vi "Mutate 1.3.3.vi"(8 "error in (no error)":errorcluster, 11 "Device Ref in":T1 format="%.0x") -> (0 "error out":errorcluster, 3 "Device Ref out":T1 format="%.0x")   [LabVIEW 2015, in "Engine Simulation Toolkit System Explorer.lvlib"]
uses:
  Engine Simulation Toolkit System Explorer.lvlib
  <vilib>/NI Veristand/Custom Device API/Custom Device Item Ref.ctl
  <vilib>/NI Veristand/Custom Device Tools/Custom Device Utility Library/NI VeriStand - Search for All Items by GUID.vi
  <vilib>/NI Veristand/Custom Device Tools/Custom Device Utility Library/NI VeriStand - Search for Item by Name.vi
  <vilib>/NI VeriStand/Custom Device Tools/Custom Device Utility Library/Custom Device Utility Library.lvlib
  <vilib>/NI VeriStand/Custom Device API/Custom Device API.lvlib
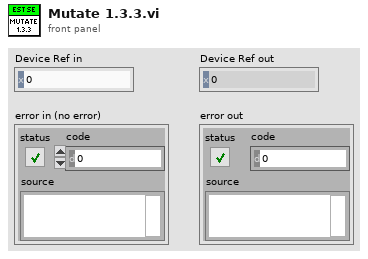
[diagram p1: front panel]
types:
  T1 = typedef "Custom Device API.lvlib/Custom Device Item Ref.ctl" = u64
  T2 = typedef "Engine Simulation Toolkit Shared.lvlib/Channel.ctl" = cluster{"Name":string, "Units":string, "Default":dbl, "Description":string, "Scalable":bool}
  T3 = cluster{"GUID.Status":string, "ChanList.Status Chans":T2[]}[]
  T4 = typedef "Custom Device API.lvlib/Custom Device Item Info.ctl" = cluster{"Name":string, "Is Channel":bool, "GUID":string, "Is Waveform":bool}
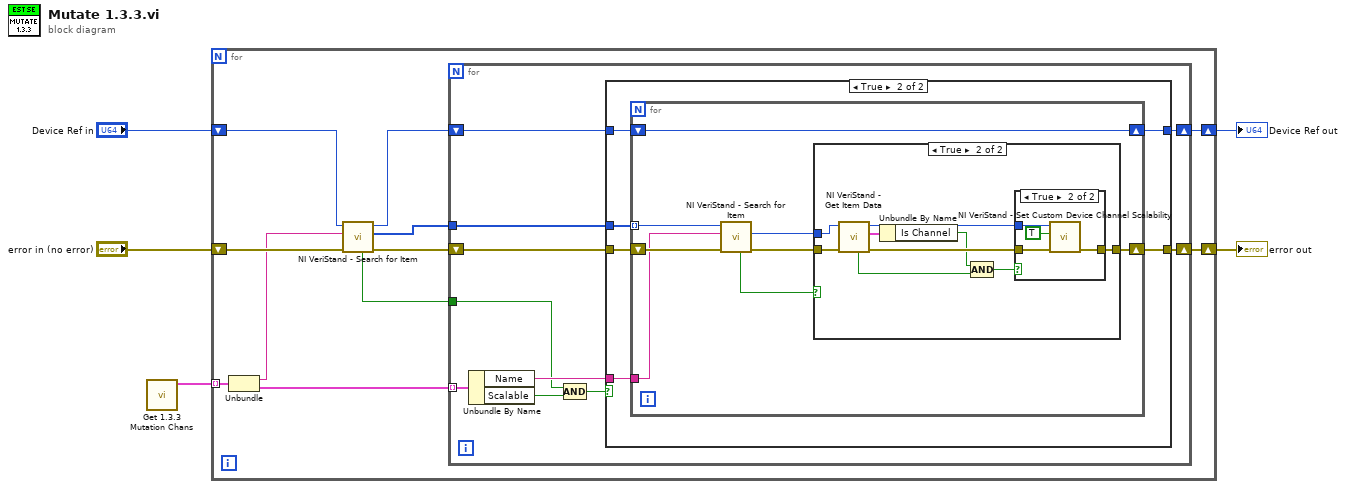
[diagram p0: block diagram]
diagram:
  n1 = call "Get 1.3.3 Mutation Chans.vi"() -> ("Array"=w1:T3)  [unwired: 11 in]
  n2 = for {
    shift-right: [w15] -> w5
    shift-left: "Device Ref in" -> [w16]
    shift-right: [w13] -> w4
    shift-left: "error in (no error)" -> [w14]
    tunnel: w1 -> [w8] mode=indexing
    n3 = Unbundle(w8) -> ("GUID.Status"=w6:string, "ChanList.Status Chans"=w7:T2[])
    n4 = call-poly <vilib>:"NI VeriStand - Search for Item.vi"("error in"=w14, "Item GUID"=w6, "Section Ref in"=w16) -> ("error out"=w9:errorcluster, "Item Refs"=w12:T1[], "Section Ref out"=w10:T1, "Found"=w11:bool)  [unwired: 5 in]
    n5 = for {
      tunnel: w7 -> [w24] mode=indexing
      tunnel: w12 -> [w22]
      tunnel: w11 -> [w18]
      shift-right: [w26] -> w15
      shift-left: w10 -> [w21]
      shift-right: [w25] -> w13
      shift-left: w9 -> [w20]
      n6 = Unbundle By Name(w24) -> ("Name"=w23:string, "Scalable"=w19:bool)
      n7 = Compound Arithmetic op=AND(w18, w19) -> (w17:bool)
      n8 = case shown="True" w17 {
        tunnel: [w28 w29] -> w26
        tunnel: w20 -> [w27 w34]
        tunnel: [w27 w33] -> w25
        tunnel: w23 -> [_ w32]
        tunnel: w22 -> [_ w31]
        tunnel: w21 -> [w28 w30]
        frame False {
        }
        frame True {
          n9 = for {
            tunnel: w32 -> [w38]
            tunnel: w31 -> [w36] mode=indexing
            shift-right: [w39] -> w33
            shift-left: w34 -> [w40]
            shift-right: [w35] -> w29
            shift-left: w30 -> [w35]
            n10 = call-poly <vilib>:"NI VeriStand - Search for Item.vi"("error in"=w40, "Item Name"=w38, "Section Ref in"=w36) -> ("error out"=w42:errorcluster, "Item Ref"=w41:T1, "Found"=w37:bool)  [unwired: 5 in, 1 out]
            n11 = case shown="True" w37 {
              tunnel: w42 -> [w43 w52]
              tunnel: w41 -> [_ w51]
              tunnel: [w43 w50] -> w39
              frame False {
              }
              frame True {
                n12 = call <vilib>:"NI VeriStand - Get Item Data.vi"("error in (no error)"=w52, "Item Ref in"=w51) -> ("error out"=w47:errorcluster, "Item Info"=w49:T4, "Item Ref out"=w48:T1, "Found"=w46:bool)  [unwired: 6 in]
                n13 = Unbundle By Name(w49) -> ("Is Channel"=w45:bool)
                n14 = Compound Arithmetic op=AND(w45, w46) -> (w44:bool)
                n15 = case shown="True" w44 {
                  tunnel: w48 -> [_ w57]
                  tunnel: w47 -> [w53 w56]
                  tunnel: [w53 w55] -> w50
                  frame False {
                  }
                  frame True {
                    n16 = call <vilib>:"NI VeriStand - Set Custom Device Channel Scalability.vi"("error in (no error)"=w56, "Scalability"=TRUE, "Channel Ref in"=w57) -> ("error out"=w55:errorcluster)  [unwired: 7 in, 1 out]
                  }
                }
              }
            }
          }
        }
      }
    }
  }
  "Device Ref out" <- w5
  "error out" <- w4
